vi "script to parameter array.vi"(11 "script":string) -> (3 "parameter array":string[](array[string]))   [LabVIEW 2020, in "Script Line.lvclass"]
uses:
  Script Line.lvclass
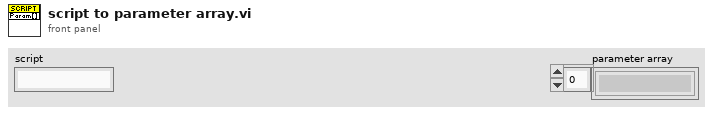
[diagram p1: front panel]
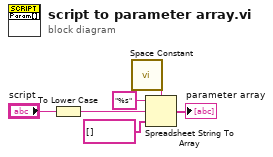
[diagram p0: block diagram]
diagram:
  n1 = To Lower Case(string="script") -> (all lower case string=w3:string)
  n2 = call <vilib>:"Space Constant.vi"() -> ("String"=w5:string)
  n3 = Spreadsheet String To Array(delimiter (Tab)=w5, format string="%s" ("포맷 문자열"), spreadsheet string=w3, array type (2D Dbl)=string[] [] ("문자열")) -> (array=→"parameter array":string[])
